vi "main 0.5.vi"() -> ()   [LabVIEW 2015]
uses:
  subvi/PHOIBOS/DEFINITIONS/DEF_dev_state.ctl
  subvi/PHOIBOS/DEFINITIONS/DEF_dev_type.ctl
  <vilib>/Utility/file.llb/Write Delimited Spreadsheet (I64).vi
  subvi/Newport ESP301/Newport ESP301.lvlib
  subvi/sp_manip.llb/sp_manip_lib.lvlib
  subvi/sp_manip.llb/tcp_gateway.lvlib
panel:
  out "appended path 2":path=path "W:/Labview/Front ends/ARPEScontrol/t0.txt"
  out "appended path":path=path "W:/Labview/Front ends/ARPEScontrol/runnumber.txt"
  out "RunNumber":u16=4
  out "# elements in queue":i32
  out "sum":dbl=3886353.0
  out "cam_fps":dbl(slide)=19.67681433793903 caption="FPS" scale=0.1..50.0
  out "max value":u32=54
  out "Intensity Graph":u32[][](graph)
  out "ESP_con?":bool=TRUE caption="ESP301"
  out "phoib_con?":bool caption="PHOIBOS"
  out "manip_con?":bool caption="manipulator"
  out "cam_con?":bool caption="camera"
  in  "main_close":bool
  in  "Tab Control":T1(tab)
  in  "ESP_delta":dbl caption="relative [mm]"
  in  "ESP_-":bool
  in  "ESP_+":bool
  in  "ESP_go":bool
  in  "ESP_dest_t":dbl caption="Delay [fs]"
  in  "ESP_dest":dbl=33.3075 caption="Position [mm]"
  in  "ESP_set_t0":bool
  in  "phoib_I_6s":dbl=3200.0
  in  "phoib_I_5s":dbl=1400.0
  in  "phoib_I_4s":dbl=4.2
  in  "phoib_I_3s":dbl
  in  "phoib_I_2s":dbl=35.0
  in  "phoib_I_1s":dbl=21.9
  in  "phoib_standby":bool
  in  "phoib_set":bool
  out "phoib_I_6":dbl caption="Screen Voltage"
  out "phoib_I_5":dbl caption="Detctor Voltage"
  out "phoib_I_4":dbl caption="Work Function"
  out "phoib_I_3":dbl caption="Coil Current"
  out "phoib_I_2":dbl caption="Pass Energy"
  out "phoib_I_1":dbl caption="Kinetic Energy"
  out "Saved Positions":string[][](table)=[["ertwertwert", "-2.299945", "-2.030214", "38.900024", "50.000762", "0.000887", "-97.998082"], ["uztgugt", "-14.999451", "-13.638894", "442.380066", "13.998380", "-1.893758", "-76.305838"], ["asdf", "-14.999451", "-13.638894", "442.380066", "13.998380", "-1.893758", "-76.305838"], ["test3", "-14.999451", "-13.638894", "441.380066", "13.998380", "-1.893758", "-76.305838"]]
  in  "Save Pos":bool
  in  "Load":bool
  in  "Delete":bool
  in  "ManipRel":dbl=1.0
  in  "ManipRel +":bool
  in  "ManipRel -":bool
  in  "manip.rel.select":enum32{"x", "y", "z", "polar", "tilt", "azimut"}(radio)=enum."polar"
  in  "Move Abs":bool
  in  "stop manip":bool
  in  "dest":dbl[](array[numeric])=[0.007141549166819264, -0.009888298846365134, 431.30615234375, 89.00040512814502, 1.109125024699864, -227.9162918846475] caption="destinations" format="%#.5g"
  out "names":string[](array[string])=["x", "y", "z", "polar", "tilt", "azimut"]
  out "pos":dbl[](array[numeric])=[0.007141549166819264, -0.009888298846365134, 431.30615234375, 89.00040512814502, 1.109125024699864, -227.9162918846475] caption="positions" format="%.5f"
  in  "Mode":T2(ring)=enum."WideAngleMode"
  in  "VoltageRange":enum16{"3.5kV", "1.5kV", "400V", "100V", "10V"}(ring)=enum."400V"
  out "ESP_pos":dbl=33.3075 caption="Position"
  out "ESP_delay":dbl caption="Delay"
  out "ESP_t0":dbl=33.3075 caption="Time Zero @"
  out "phoib_I_7":dbl caption="Conversion Voltage"
  in  "phoib_I_7s":dbl
  in  "phoib_I_8s":dbl
  in  "phoib_I_9s":dbl
  out "phoib_I_8":dbl caption="FD1"
  out "phoib_I_9":dbl caption="FD2"
  out "electronics temp [°C]":i32=30
  out "CCD temp [°C]":i32=-13
  in  "gain":bool
  in  "exposure [ms]":u32=20
  in  "binning":u16(ring)=2 items=["X 1", "X 2", "X 4", "X 8"]
  in  "cam_dark?":bool caption="subtract dark?"
  in  "cam_dark":bool
  in  "cam_dark#":u32 max=1000
  in  "cam_burst":bool
  in  "cam_burstnr":u32 max=100000
  out "cam_burst_progress":i32(slide) scale=0.0..500.0
  in  "delscan_picspstep":u16=1 caption="pics/step" min=1 step=1
  in  "delscan_abort":bool
  out "delscan_progress":u32(slide) scale=0.0..20.0
  in  "delscan_go":bool
  out "delscan_pos":dbl caption="current delay [fs]"
  in  "delscan_end":dbl caption="end [fs]"
  in  "delscan_stepsize":dbl caption="stepsize [fs]"
  in  "delscan_start":dbl caption="start [fs]"
  in  "comment":string
  in  "Radio Buttons":enum32{"Radio Selection 1", "Radio Selection 2"}(radio)
  out "opti_frames":dbl=25.0 caption="#steps_opti"
  out "opti_current_frame":i32=25
  out "Measurement Progress":u8(slide) scale=0.0..100.0
  out "Camera Aquisition":u8(slide) scale=0.0..100.0
  in  "Optimize":bool
  in  "OptiStepSize":dbl=-1.0 caption="Step Size"
  in  "OptiRange":dbl=25.0 caption="Range"
  in  "meas_axis":string(combo)="tilt" caption="Axis"
  in  "meas_avg":i32=60 caption="Frames2Average"
  in  "OptiCancel":bool
  out "#steps_opti":dbl=25.0
  out "current_step_opti":i32=25
  out "ETA":string
  in  "BasePath":path=path "Z:/PESdata"
  in  "Path":path=path "Z:/software/ManipulatorControl/save.txt"
  in  "ROI Bottom":i32=32
  in  "ROI Top":i32=1
  in  "ROI Right":i32=40
  in  "ROI Left":i32=1
  in  "ESP Axis":i32=1 min=1 max=3
  in  "manip_init":bool
  in  "manip_release":bool
  in  "phoib_init":bool
  in  "phoib_release":bool
  in  "ESP_init":bool
  in  "ESP_release":bool
  in  "ESP301 VISA":refnum<visa-resource-name>="COM8"
  in  "cam_boardnr":i32
  in  "cam_init":bool
  in  "cam_release":bool
  out "error out":errorcluster
  out "error out 2":errorcluster
  out "state":T3 items=["Off"=-1, "Standby"=0, "On"=1]
  # "step _ of _"
  # "step _ of _"
  # "manip"
  # "phoib"
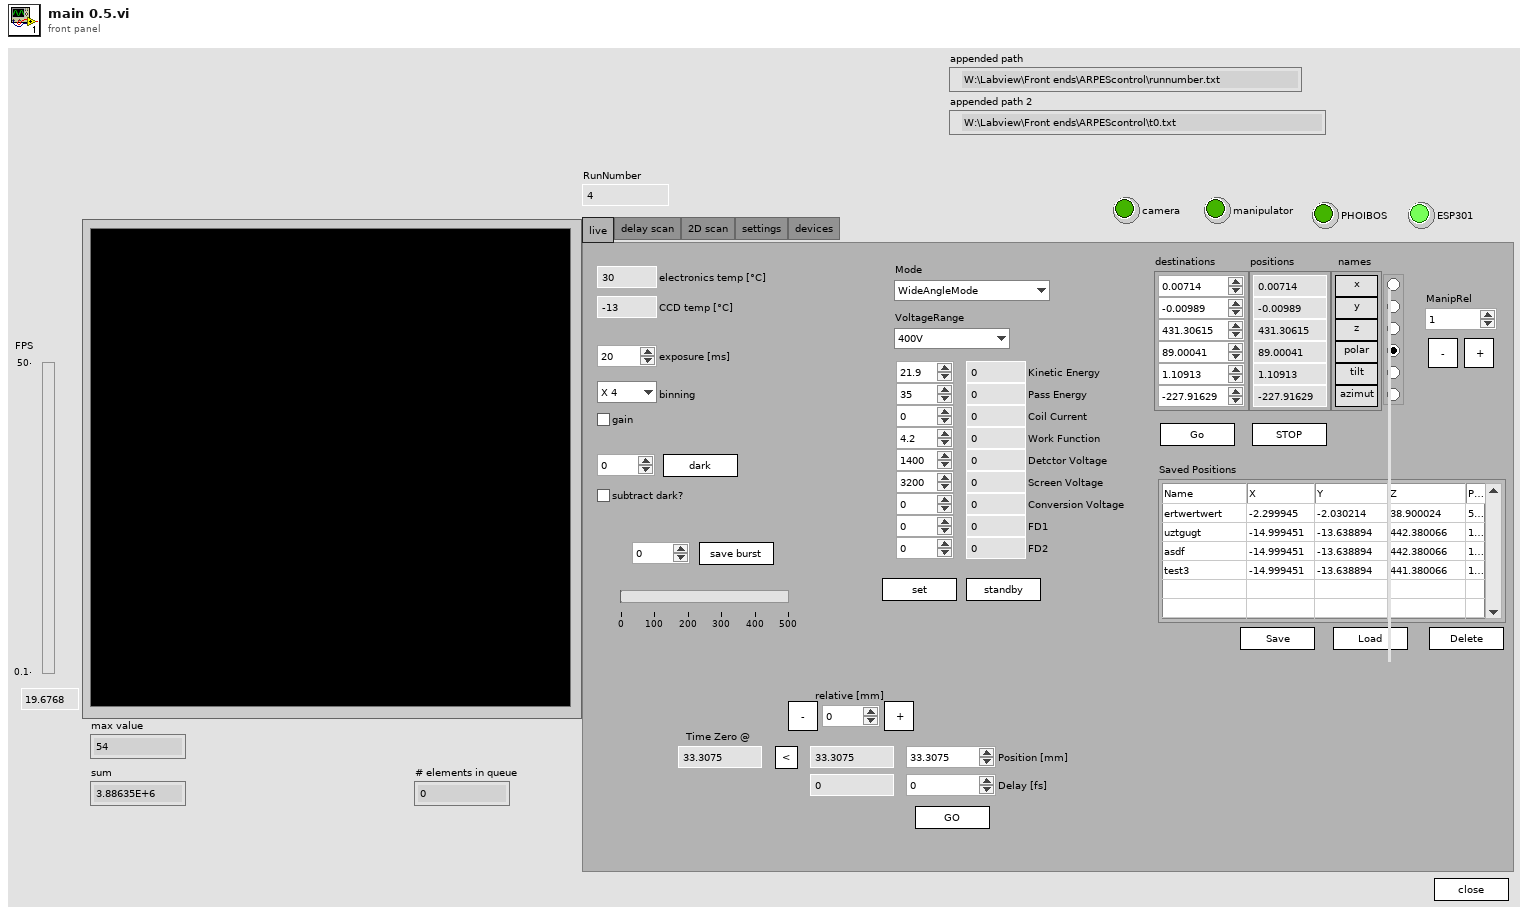
[diagram p1: front panel]
types:
  T1 = enum32{"live", "delay scan", "2D scan", "settings", "devices"}
  T2 = enum16{"HighMagnification", "MediumMagnification", "LowMagnification", "HighAngularDispersion", "MediumAngularDispersion", "LowAngularDispersion", "WideAngleMode", "LargeArea", "MediumArea", "SmallArea", "HighMagnification2", "SmallArea2", "ImagingMode"}
  T3 = typedef "DEF_dev_state.ctl" = i32
  T4 = cluster{"Camera type":u32, "Operating mode\nHP & QE / HS & DiCam Pro ":u32, "Frame trigger \n(High Performance and QE only)":u16, "Sequence trigger":u16, "Low Light\n(QE only)":bool, "Gain":bool, "Horzontal\nbinning":u16, "Vertical\nbinning ":u16, "ROI Left":i32, "ROI Right":i32, "ROI Top":i32, "ROI Bottom":i32}
  T5 = enum16{"open", "replace", "create", "open or create", "replace or create", "replace or create with confirmation"}
  T6 = cluster{"Axis_Name":string, "Axis_Type":string, "Axis_Position":dbl, "continous":bool, "moving":bool}[]
  T7 = cluster{"Axis_Name":string, "Axis_Type":string, "Axis_Position":dbl, "continous":bool, "moving":bool}
  T8 = typedef "DEF_dev_type.ctl" = enum32{"devA (analyzer)", "devD (detector)"}
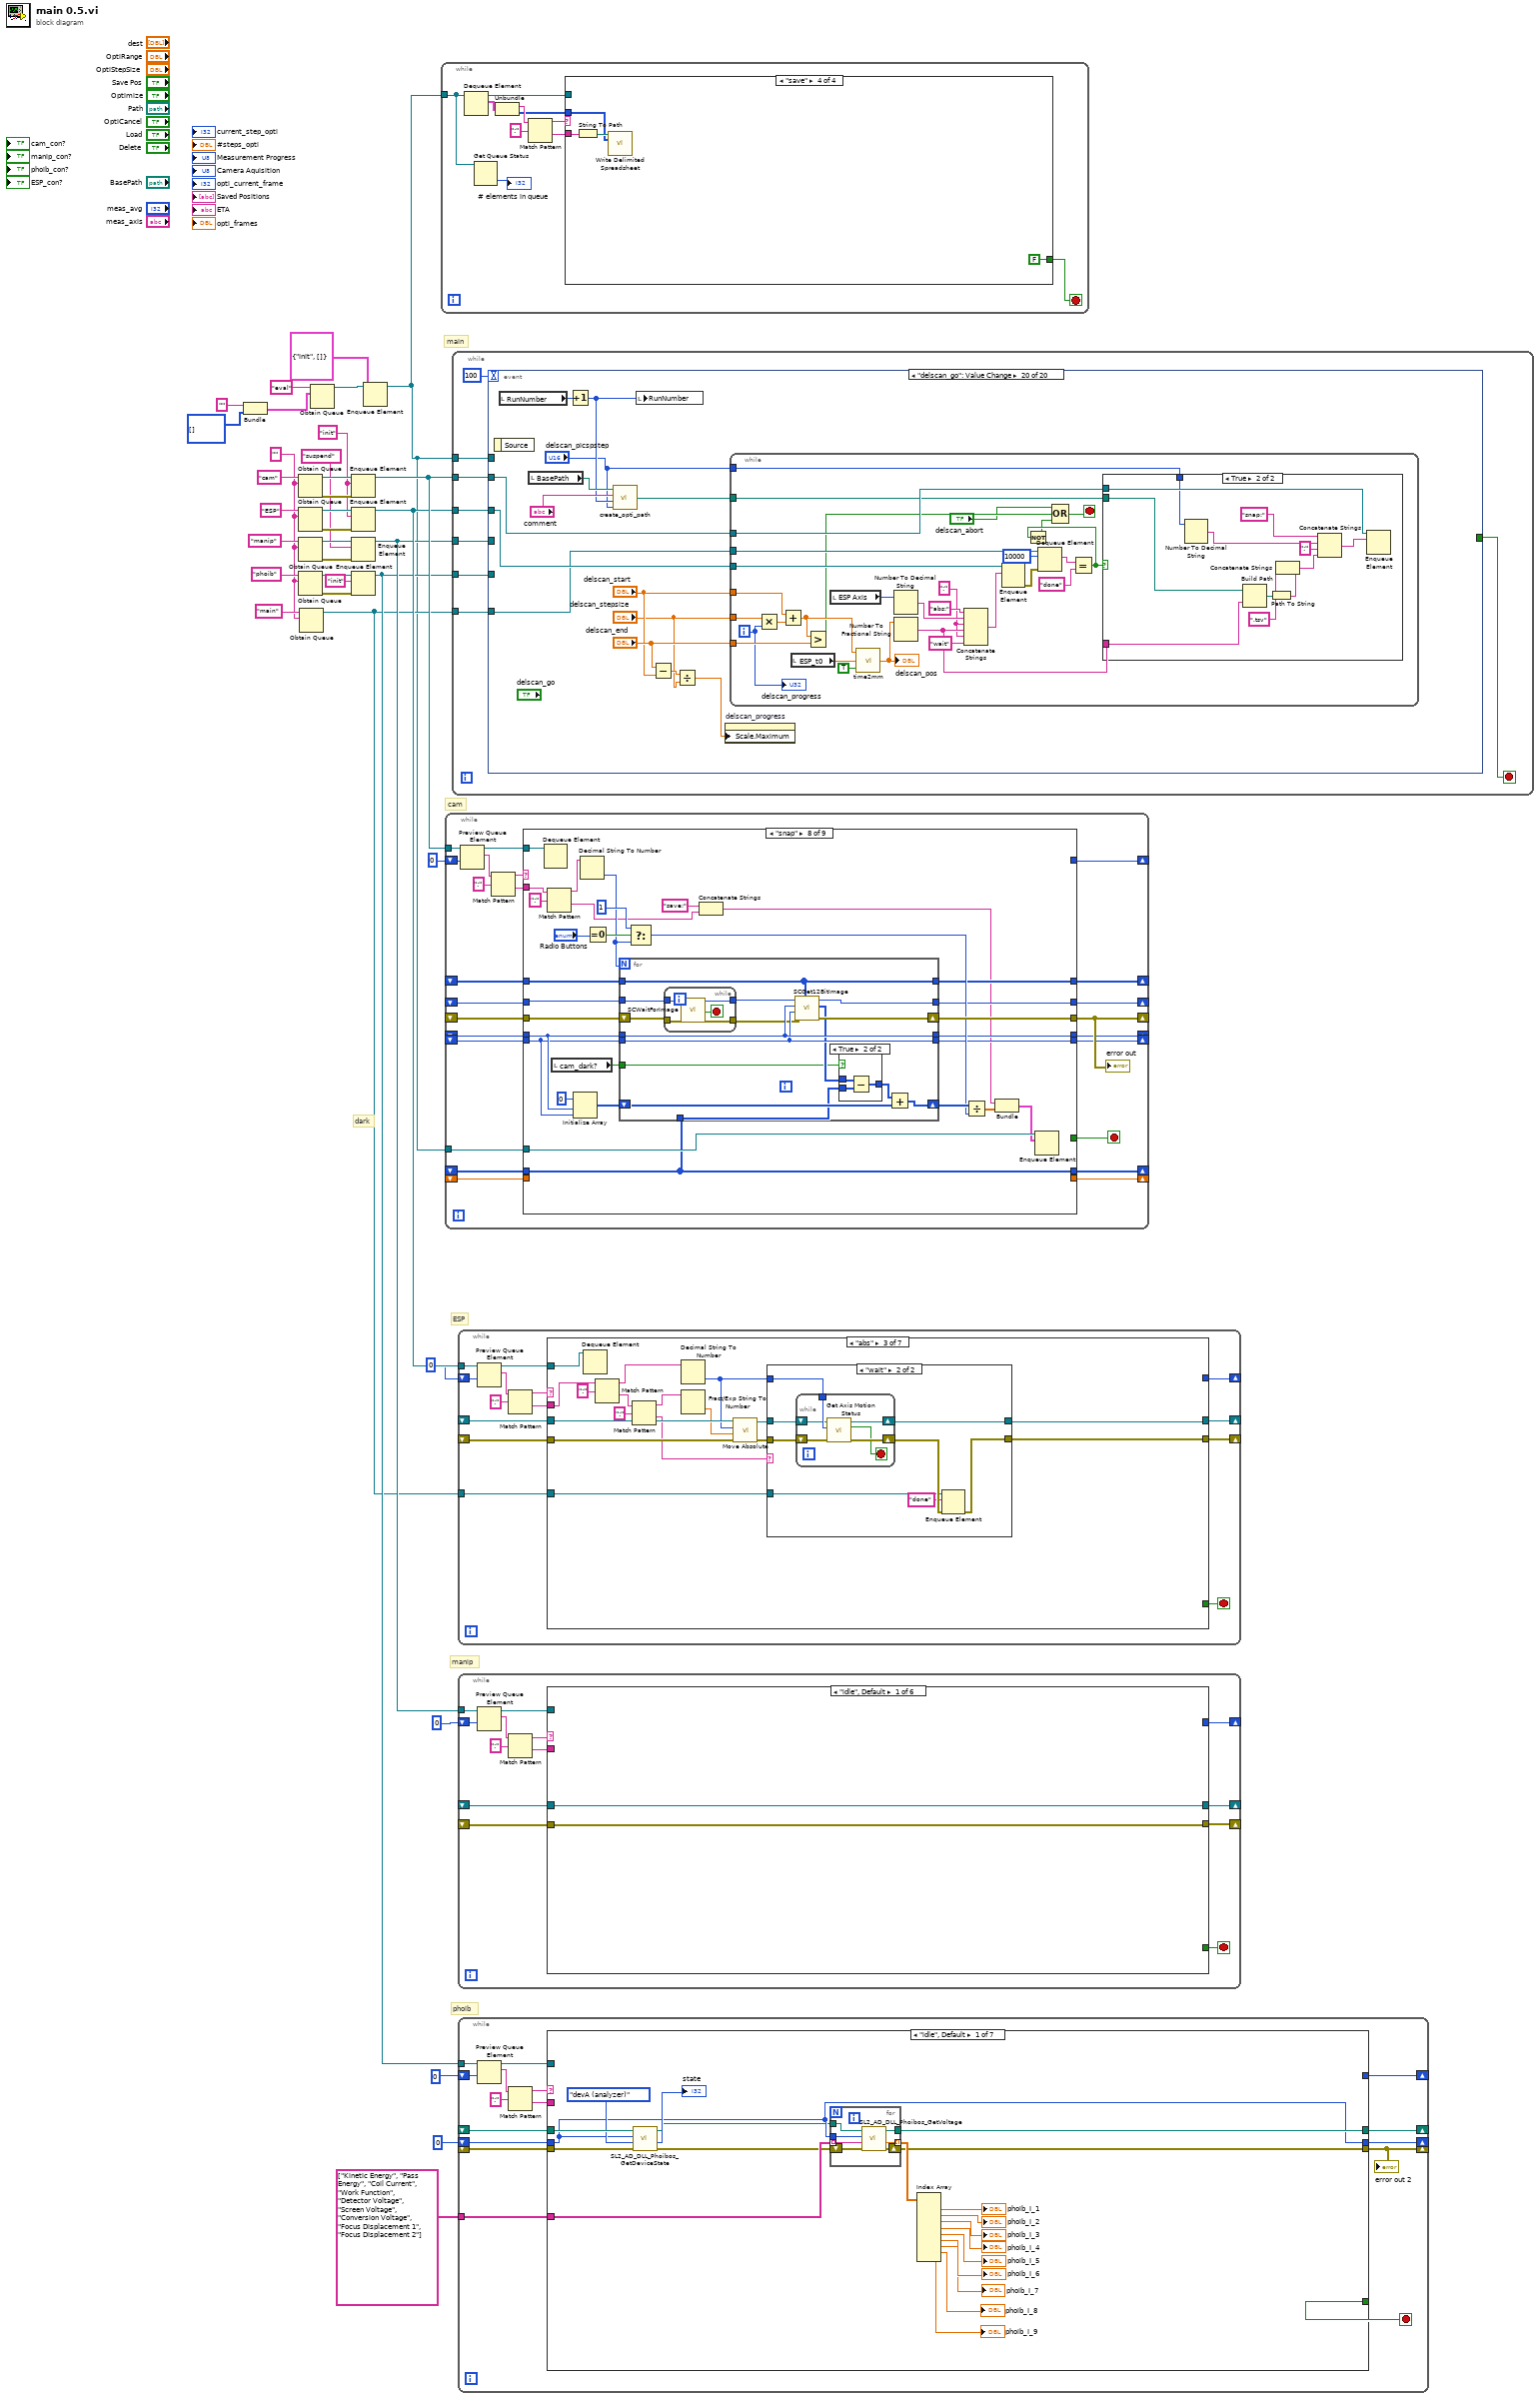
[diagram p0: block diagram]
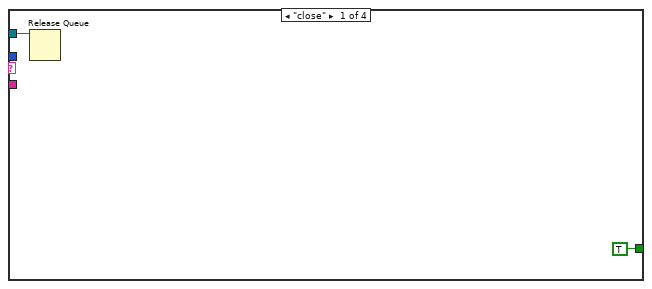
[diagram p2: hidden frame]
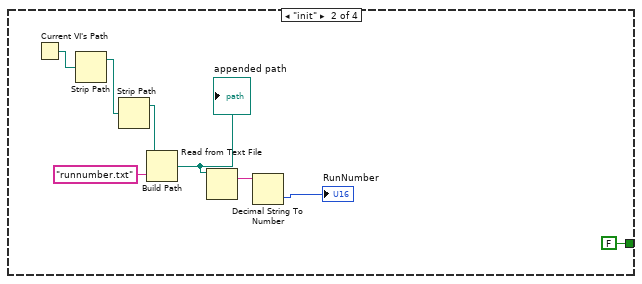
[diagram p3: hidden frame]
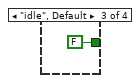
[diagram p4: hidden frame]
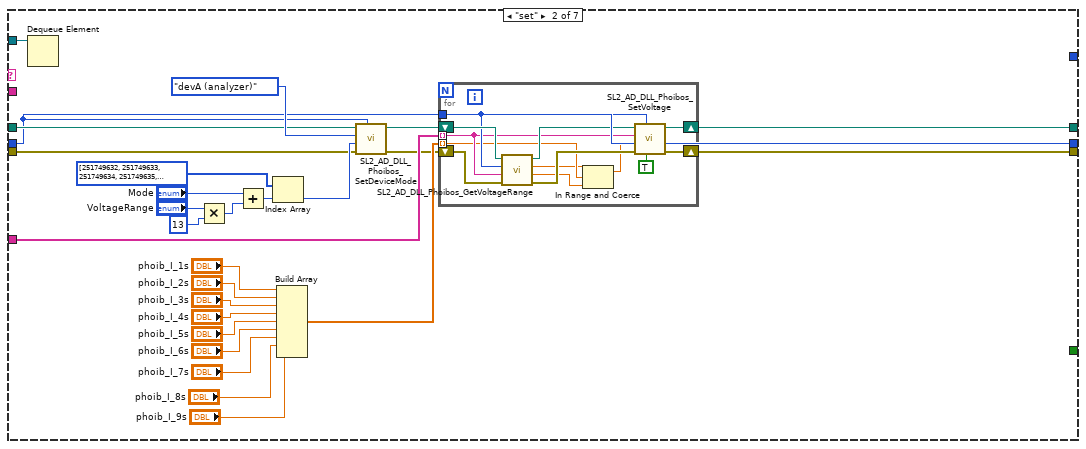
[diagram p5: hidden frame]
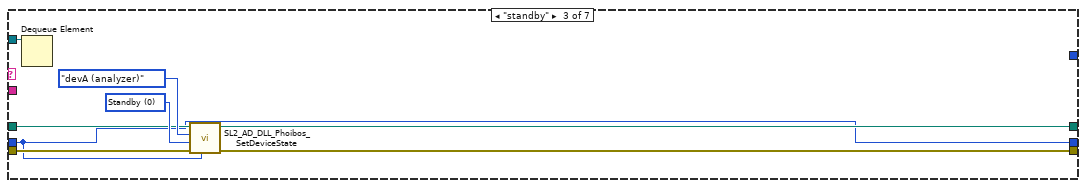
[diagram p6: hidden frame]
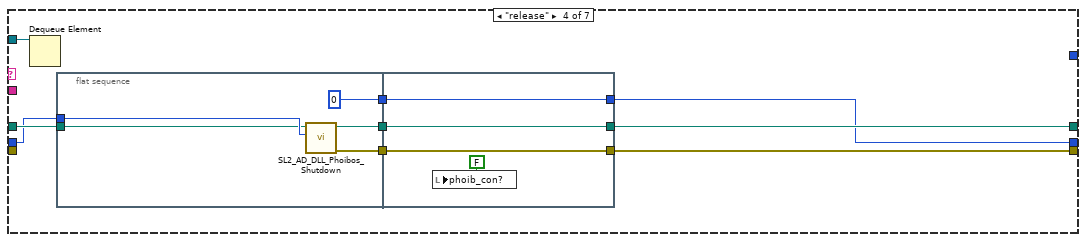
[diagram p7: hidden frame]
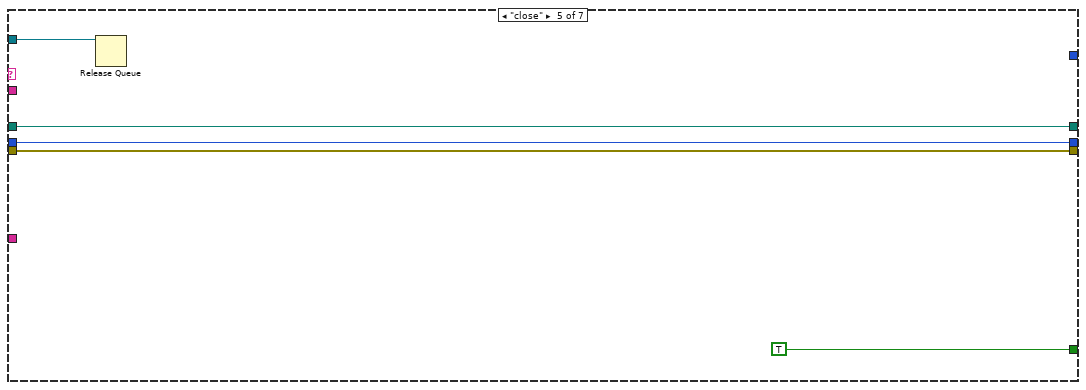
[diagram p8: hidden frame]
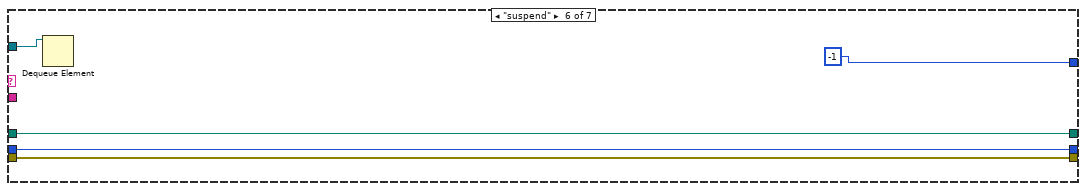
[diagram p9: hidden frame]
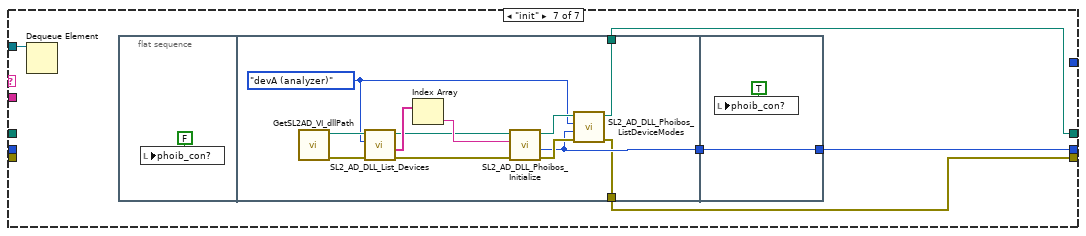
[diagram p10: hidden frame]
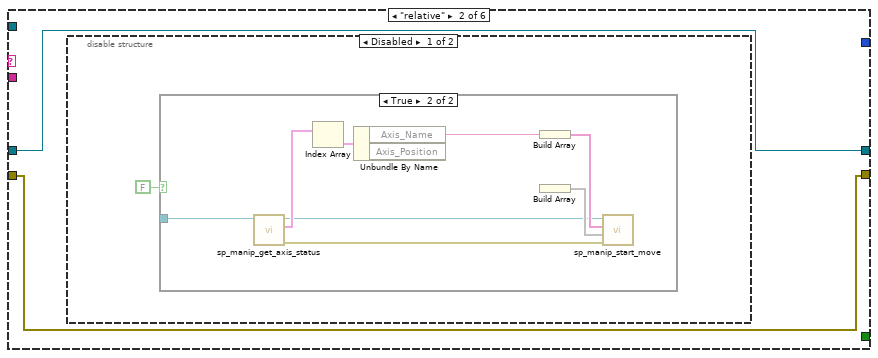
[diagram p11: hidden frame]
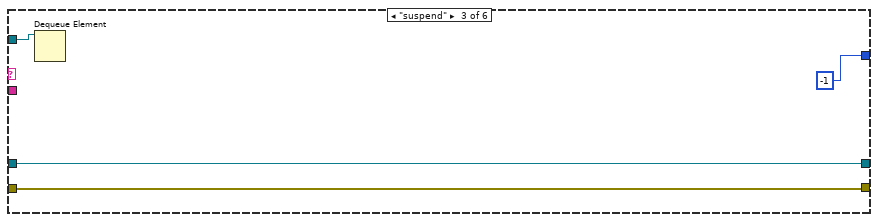
[diagram p14: hidden frame]
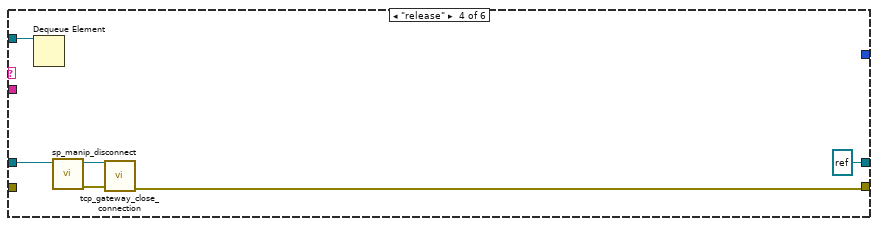
[diagram p15: hidden frame]
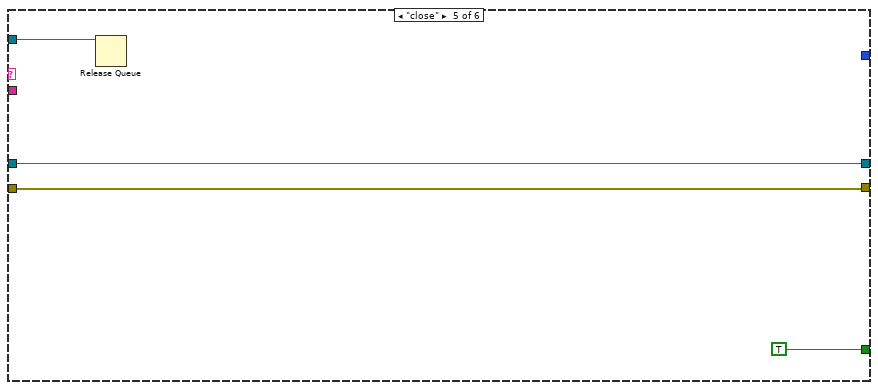
[diagram p16: hidden frame]
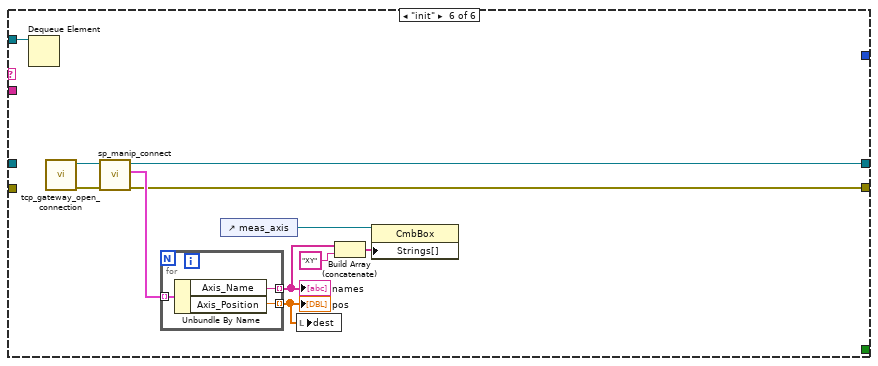
[diagram p17: hidden frame]
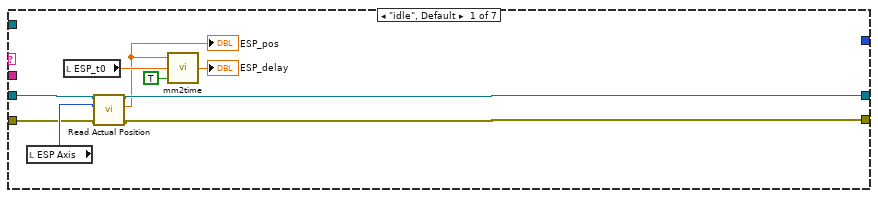
[diagram p18: hidden frame]
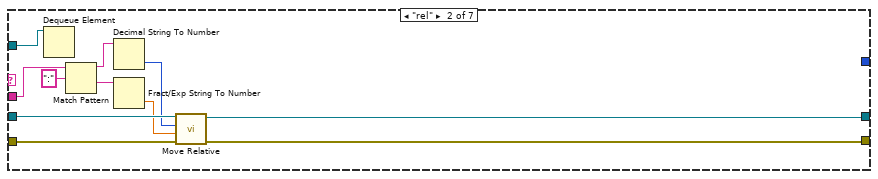
[diagram p19: hidden frame]
diagram:
  w4 = "init" ("name (unnamed)")
  w9 = "" ("name (unnamed)")
  # "dark"
  # "phoib"
  # "manip"
  # "ESP"
  # "cam"
  # "main"
  n1 = Bundle("", u32[][] []) -> (w7:cluster{string, u32[][]})  [unwired: 1 in]
  n2 = Obtain Queue(name (unnamed)="cam", element data type=w9) -> (queue out=w34:refnum<queue>, error out=w33:errorcluster)  [unwired: 3 in, 1 out]
  n3 = Obtain Queue(name (unnamed)="ESP", element data type=w9) -> (queue out=w30:refnum<queue>, error out=w31:errorcluster)  [unwired: 3 in, 1 out]
  n4 = Obtain Queue(name (unnamed)="manip", element data type=w9) -> (queue out=w27:refnum<queue>, error out=w26:errorcluster)  [unwired: 3 in, 1 out]
  n5 = Obtain Queue(name (unnamed)="phoib", element data type=w9) -> (queue out=w24:refnum<queue>, error out=w25:errorcluster)  [unwired: 3 in, 1 out]
  n6 = Obtain Queue(name (unnamed)="main", element data type=w9) -> (queue out=w10:refnum<queue>)  [unwired: 3 in, 2 out]
  n7 = Obtain Queue(name (unnamed)="eval", element data type=w7) -> (queue out=w3:refnum<queue>)  [unwired: 3 in, 2 out]
  n8 = Enqueue Element(queue=w34, element=w4, error in (no error)=w33) -> (queue out=w32:refnum<queue>)  [unwired: 1 in, 2 out]
  n9 = Enqueue Element(queue=w30, element=w4, error in (no error)=w31) -> (queue out=w21:refnum<queue>)  [unwired: 1 in, 2 out]
  n10 = Enqueue Element(queue=w27, element="suspend" ("name (unnamed)"), error in (no error)=w26) -> (queue out=w20:refnum<queue>)  [unwired: 1 in, 2 out]
  n11 = Enqueue Element(queue=w24, element="init", error in (no error)=w25) -> (queue out=w19:refnum<queue>)  [unwired: 1 in, 2 out]
  n12 = Enqueue Element(queue=w3, element=cluster{string, u32[][]} {"init", []}) -> (queue out=w2:refnum<queue>)  [unwired: 2 in, 2 out]
  n13 = while {
    tunnel: w2 -> [w37]
    stop <- w38 stop-if-true
    n14 = Dequeue Element(queue=w37) -> (queue out=w43:refnum<queue>, element=w42:cluster{string, u32[][]})  [unwired: 2 in, 2 out]
    n15 = Get Queue Status(queue=w37) -> (# elements in queue=→"# elements in queue":i32)  [unwired: 2 in, 7 out]
    n16 = Unbundle(w42) -> (w41:string, w40:u32[][])
    n17 = Match Pattern(string=w41, regular expression=":") -> (before substring=w44:string, after substring=w39:string)  [unwired: 1 in, 2 out]
    n18 = case shown="\"save\"" w44 {
      tunnel: w43 -> [w47 _ _ _]
      tunnel: w40 -> [_ _ _ w58]
      tunnel: w39 -> [_ _ _ w60]
      tunnel: [TRUE FALSE FALSE FALSE] -> w38
      frame "close" {
        n19 = Release Queue(queue=w47) -> ()  [unwired: 2 in, 3 out]
      }
      frame "init" {
        n20 = Current VI's Path() -> (path=w55:path)
        n21 = Strip Path(path=w55) -> (stripped path=w49:path)  [unwired: 1 out]
        n22 = Strip Path(path=w49) -> (stripped path=w48:path)  [unwired: 1 out]
        n23 = Build Path(base path=w48, name or relative path="runnumber.txt") -> (appended path=w53:path)
        "appended path" <- w53
        n24 = Read from Text File(file (use dialog)=w53) -> (text=w52:string)  [unwired: 3 in, 3 out]
        n25 = Decimal String To Number(string=w52) -> (number=→"RunNumber":i32)  [unwired: 2 in, 1 out]
      }
      frame "idle", Default {
      }
      frame "save" {
        n26 = String To Path(string=w60) -> (path=w59:path)
        n27 = call-poly <vilib>:"Write Delimited Spreadsheet.vi"("file path (dialog if empty)"=w59, "2D data"=w58) -> ()  [unwired: 12 in, 2 out]
      }
    }
  }
  n28 = while {
    tunnel: w32 -> [w84]
    shift-right: [w78] -> _
    shift-left: _ -> [w77]
    shift-right: [w76] -> _
    shift-left: _ -> [w72]
    shift-right: [w75] -> _
    shift-left: _ -> [w71]
    shift-right: [w74] -> _
    shift-left: _ -> [w70]
    shift-right: [w73] -> _
    shift-left: _ -> [w69]
    shift-right: [w66] -> _
    shift-left: 0 -> [w67]
    shift-right: [w65] -> _
    shift-left: _ -> [w64]
    shift-right: [w63] -> _
    shift-left: _ -> [w62]
    tunnel: w2 -> [w61]
    stop <- w68 stop-if-true
    n29 = Preview Queue Element(queue=w84, timeout in ms (-1)=w67) -> (queue out=w83:refnum<queue>, element=w82:string)  [unwired: 1 in, 2 out]
    n30 = Match Pattern(string=w82, regular expression=":") -> (before substring=w79:string, after substring=w80:string)  [unwired: 1 in, 2 out]
    n31 = case shown="\"snap\"" w79 {
      tunnel: w83 -> [w93 w121 w151 w205 w217 _ w257 w286 w346]
      tunnel: w80 -> [_ _ w159 _ _ _ _ w290 _]
      tunnel: [w87 w110 w148 w204 w215 w241 w255 w302 w344] -> w78
      tunnel: w77 -> [_ _ w156 w204 w215 w241 w262 w310 w344]
      tunnel: [w92 w122 w149 u64 0 ("Hout") w214 w232 w261 w299 w343] -> w76
      tunnel: [w94 w123 w150 w199 w213 w235 w256 w309 w342] -> w75
      tunnel: [w86 w114 w147 w203 w212 w240 w254 w301 w341] -> w74
      tunnel: [w86 w113 w146 w202 w211 w239 w253 w300 w340] -> w73
      tunnel: w72 -> [_ w125 w155 w201 w214 w231 w263 w285 w343]
      tunnel: w71 -> [_ w124 w152 _ w213 w230 w260 w313 w342]
      tunnel: w70 -> [_ _ w154 w203 w212 w240 w259 w308 w341]
      tunnel: w69 -> [_ _ w153 w202 w211 w239 w258 w307 w340]
      tunnel: [_ _ _ _ TRUE _ _ _ _] -> w68
      tunnel: [_ _ _ _ _ _ _ _ -1] -> w66
      tunnel: [w85 w107 _ _ _ w227 _ _ _] -> w65
      tunnel: w64 -> [w85 w107 _ _ _ w226 _ _ _]
      tunnel: [w87 w109 w145 w197 w210 w221 w251 w293 w339] -> w63
      tunnel: w62 -> [_ w109 w145 w197 w210 w221 _ w293 w339]
      tunnel: w61 -> [_ _ w143 _ _ _ _ w298 _]
      frame "init" {
        w86 = 0 ("Horizontal size")
        w87 = u16[][] []
        n32 = flat-sequence {
          tunnel: [w96] -> w91
          tunnel: [w97] -> w90
          tunnel: [w105] -> w92
          tunnel: [w106] -> w94
          tunnel: w91 -> [w106]
          tunnel: w90 -> [w105]
          frame #0 {
            n33 = local write "cam_con?"(FALSE ("cam_con?")) -> ()
          }
          frame #1 {
            n34 = call "SCInitBoard.vi"("boardnr"="cam_boardnr") -> ("Hout"=w100:u32, "error out"=w101:errorcluster)  [unwired: 1 in, 1 out]
            n35 = call "SCSetupCamera.vi"("Handle"=w100, "error in (no error)"=w101) -> ("Hout"=w102:u64, "error out"=w103:errorcluster)  [unwired: 1 out]
            n36 = call "SCStopCOC.vi"("error in (no error)"=w103, "Stop mode"=0, "Handle"=w102) -> ("error out"=w96:errorcluster, "Hout"=w97:u64)
          }
          frame #2 {
            n37 = local write "cam_con?"(TRUE ("cam_con?")) -> ()
          }
        }
        n38 = Dequeue Element(queue=w93) -> (queue out=w89:refnum<queue>)  [unwired: 2 in, 3 out]
        n39 = Enqueue Element At Opposite End(queue=w89, element="set") -> ()  [unwired: 2 in, 3 out]
      }
      frame "set" {
        w120 = u32 1 ("Operating mode\nHP & QE / HS & DiCam Pro")
        n40 = Dequeue Element(queue=w121) -> ()  [unwired: 2 in, 4 out]
        n41 = Bundle By Name(cluster=cluster{"Delay":dbl, "Exposure ":dbl} {"Delay"=0.0, "Exposure "=0.0} ("Delay and exposure"), "Exposure"="exposure [ms]") -> (w117:cluster{"Delay":dbl, "Exposure ":dbl})
        n42 = call "SCStopCOC.vi"("error in (no error)"=w124, "Stop mode"=0, "Handle"=w125) -> ("error out"=w140:errorcluster, "Hout"=w139:u64)
        n43 = Bundle By Name(cluster=T4 {"Camera type"=0, "Operating mode\nHP & QE / HS & DiCam Pro "=0, "Frame trigger \n(High Performance and QE only)"=0, "Sequence trigger"=0, "Low Light\n(QE only)"=FALSE, "Gain"=FALSE, "Horzontal\nbinning"=0, "Vertical\nbinning "=0, "ROI Left"=1, "ROI Right"=20, "ROI Top"=1, "ROI Bottom"=15} ("Camera controls"), "Operating mode\nHP & QE / HS & DiCam Pro"=w120, "Horzontal\nbinning"="binning", "Vertical\nbinning"="binning", "ROI Left"="ROI Left", "ROI Right"="ROI Right", "ROI Top"="ROI Top", "ROI Bottom"="ROI Bottom", "Gain"="gain") -> (w135:T4)
        n44 = call "New delay and exposure forma.vi"("Operating mode\nHP & QE / HS & DiCam Pro"=w120, "Delay and exposure"=w117) -> ("Output table"=w136:string)  [unwired: 3 in]
        n45 = call "SCSetCoC.vi"("error in (no error)"=w140, "Delay and exposure table"=w136, "Camera controls"=w135, "Handle"=w139) -> ("error out"=w128:errorcluster, "Hout"=w127:u64)  [unwired: 1 out]
        n46 = call "SCGetImageSize.vi"("Handle"=w127, "error in (no error)"=w128) -> ("Hout"=w126:u64, "error out"=w108:errorcluster, "Horizontal size"=w114:i32, "Vertical size"=w113:i32)  [unwired: 2 out]
        n47 = Greater?(x=w114, y=w113) -> (0:w115:bool)
        n48 = Initialize Array(u16 0 ("dimension size"), w113, w114) -> (w110:u16[][])
        n49 = call "SCRun.vi"("error in (no error)"=w108, "Run mode"=0, "Handle"=w126) -> ("error out"=w123:errorcluster, "Hout"=w122:u64)  [unwired: 1 out]
        n50 = Select(t=w114, s=w115, f=w113) -> (s? t:f=w112:i32)
        n51 = property on="Intensity Graph" class="IntGraph (strict)"("XScale.Maximum"=w112, "YScale.Maximum"=w112) -> ()  [unwired: 2 in, 2 out]
      }
      frame "burst" {
        n52 = Match Pattern(string=w159, regular expression=":") -> (before substring=w158:string, after substring=w157:string)  [unwired: 1 in, 2 out]
        n53 = Dequeue Element(queue=w151) -> ()  [unwired: 2 in, 4 out]
        n54 = String To Path(string=w157) -> (path=w141:path)
        n55 = Decimal String To Number(string=w158) -> (number=w144:i32)  [unwired: 2 in, 1 out]
        n56 = property on="cam_burst_progress" class="Slide (strict)"("Scale.Maximum"=w144) -> ()  [unwired: 2 in, 2 out]
        n57 = for {
          N: w144 -> [_]
          tunnel: w156 -> [w177]
          tunnel: w155 -> [w186]
          tunnel: w154 -> [w176]
          tunnel: w153 -> [w175]
          tunnel: w145 -> [w181]
          tunnel: [w179] -> w149
          shift-right: [w178] -> w150
          shift-left: w152 -> [w185]
          tunnel: [w177] -> w148
          tunnel: [w176] -> w147
          tunnel: [w175] -> w146
          tunnel: w143 -> [w174]
          tunnel: 100000 ("x") -> [w167]
          tunnel: w141 -> [w166]
          i -> [w161]
          w187 = 0 items=["Normal", "Upside down"] ("mode")
          n58 = Add(x=w167, y=w161) -> (x+y=w171:i32)
          n59 = while {
            tunnel: [w195] -> w183
            tunnel: [w194] -> w184
            tunnel: w186 -> [w193]
            tunnel: w185 -> [w192]
            stop <- w196 stop-if-true
            n60 = call "SCWaitForImage.vi"("Handle"=w193, "error in (no error)"=w192) -> ("Hout"=w194:u64, "Image Valid"=w196:bool, "error out"=w195:errorcluster)  [unwired: 15 in]
          }
          n61 = Number To Decimal String(number=w171) -> (decimal integer string=w170:string)  [unwired: 1 in]
          n62 = String Subset(string=w170, offset (0)=1) -> (substring=w168:string)  [unwired: 1 in]
          n63 = local read "cam_dark?"() -> (w180:bool)
          n64 = Build Path(base path=w166, name or relative path=w168) -> (appended path=w165:path)
          n65 = call "SCGet12BitImage.vi"("mode"=w187, "Input array"=w177, "error in (no error)"=w183, "Vertical size"=w175, "Horizontal size"=w176, "Handle"=w184) -> ("error out"=w178:errorcluster, "imgdata"=w182:u16[][], "Hout"=w179:u64)  [unwired: 1 in]
          n66 = Path To String(path=w165) -> (string=w164:string)
          n67 = Concatenate Strings("save:" ("string"), w164) -> (w163:string)
          n68 = case shown="True" w180 {
            tunnel: w182 -> [w188 w191]
            tunnel: w181 -> [_ w190]
            tunnel: [w188 w189] -> w162
            frame False {
            }
            frame True {
              n69 = Subtract(x=w191, y=w190) -> (x-y=w189:u32[][])
            }
          }
          n70 = local write "Intensity Graph"(w162) -> ()
          n71 = Bundle(w163, "imgdata"=w162) -> (w173:cluster{string, "imgdata":u32[][]})  [unwired: 1 in]
          n72 = Enqueue Element(queue=w174, element=w173) -> ()  [unwired: 2 in, 3 out]
          "cam_burst_progress" <- w161
        }
      }
      frame "release" {
        n73 = Dequeue Element(queue=w205) -> ()  [unwired: 2 in, 4 out]
        n74 = flat-sequence {
          tunnel: w201 -> [w207]
          tunnel: [w206] -> w198
          tunnel: [w209] -> w199
          tunnel: w198 -> [w209]
          frame #0 {
            n75 = call "SCCloseBoard.vi"("Handle"=w207) -> ("error out"=w206:errorcluster)  [unwired: 1 in, 2 out]
          }
          frame #1 {
            n76 = local write "cam_con?"(FALSE ("cam_con?")) -> ()
          }
        }
      }
      frame "close" {
        n77 = Release Queue(queue=w217) -> ()  [unwired: 2 in, 3 out]
      }
      frame "idle", Default {
        w238 = 0 items=["Normal", "Upside down"] ("mode")
        n78 = call <vilib>:"High Resolution Relative Seconds.vi"() -> ("relative seconds"=w227:dbl)
        n79 = while {
          tunnel: [w249] -> w228
          tunnel: [w248] -> w229
          tunnel: w231 -> [w247]
          tunnel: w230 -> [w246]
          stop <- w250 stop-if-true
          n80 = call "SCWaitForImage.vi"("Handle"=w247, "error in (no error)"=w246) -> ("Hout"=w248:u64, "Image Valid"=w250:bool, "error out"=w249:errorcluster)  [unwired: 15 in]
        }
        n81 = Subtract(x=w227, y=w226) -> (x-y=w225:dbl)
        n82 = Reciprocal(x=w225) -> (1/x=→"cam_fps":dbl)
        n83 = call "SCGet12BitImage.vi"("mode"=w238, "Input array"=w241, "error in (no error)"=w228, "Vertical size"=w239, "Horizontal size"=w240, "Handle"=w229) -> ("error out"=w236:errorcluster, "imgdata"=w222:u16[][], "Hout"=w237:u64)  [unwired: 1 in]
        n84 = case shown="True" "cam_dark?" {
          tunnel: w222 -> [w242 w245]
          tunnel: w221 -> [_ w244]
          tunnel: [w242 w243] -> w219
          frame False {
          }
          frame True {
            n85 = Subtract(x=w245, y=w244) -> (x-y=w243:u32[][])
          }
        }
        "Intensity Graph" <- w219
        n86 = call "SCGetStatus.vi"("Handle"=w237, "error in (no error)"=w236) -> ("Hout"=w232:u64, "Electronics temperature"=→"electronics temp [°C]":i32, "CCD temperature"=→"CCD temp [°C]":i32, "error out"=w235:errorcluster)  [unwired: 2 out]
        n87 = Array Max & Min(array=w219) -> (max value=→"max value":u32)  [unwired: 3 out]
        n88 = Add Array Elements(numeric array=w219) -> (sum=→"sum":u32)
      }
      frame "dark" {
        n89 = Dequeue Element(queue=w257) -> ()  [unwired: 2 in, 4 out]
        n90 = Initialize Array(u32 0, w258, w259) -> (w266:u32[][])
        n91 = for {
          N: "cam_dark#" -> [_]
          tunnel: w259 -> [w269]
          tunnel: w258 -> [w268]
          tunnel: w262 -> [w270]
          shift-right: [w275] -> w265
          shift-left: w266 -> [w276]
          tunnel: w263 -> [w274]
          tunnel: [w272] -> w261
          shift-right: [w271] -> w256
          shift-left: w260 -> [w273]
          tunnel: [w270] -> w255
          tunnel: [w269] -> w254
          tunnel: [w268] -> w253
          n92 = while {
            tunnel: [w283] -> w278
            tunnel: [w282] -> w279
            tunnel: w274 -> [w281]
            tunnel: w273 -> [w280]
            stop <- w284 stop-if-true
            n93 = call "SCWaitForImage.vi"("Handle"=w281, "error in (no error)"=w280) -> ("Hout"=w282:u64, "Image Valid"=w284:bool, "error out"=w283:errorcluster)  [unwired: 15 in]
          }
          n94 = call "SCGet12BitImage.vi"("Input array"=w270, "error in (no error)"=w278, "Vertical size"=w268, "Horizontal size"=w269, "Handle"=w279) -> ("error out"=w271:errorcluster, "imgdata"=w277:u16[][], "Hout"=w272:u64)  [unwired: 2 in]
          n95 = Add(x=w277, y=w276) -> (x+y=w275:u32[][])
        }
        n96 = Divide(x=w265, y="cam_dark#") -> (x/y=w252:dbl[][])
        n97 = To Unsigned Long Integer(number=w252) -> (unsigned 32bit integer=w251:u32[][])
      }
      frame "snap" {
        n98 = Dequeue Element(queue=w286) -> ()  [unwired: 2 in, 4 out]
        n99 = Match Pattern(string=w290, regular expression=":") -> (before substring=w289:string, after substring=w287:string)  [unwired: 1 in, 2 out]
        n100 = local read "cam_dark?"() -> (w292:bool)
        n101 = Initialize Array(u32 0 ("element"), w308, w307) -> (w312:u32[][])
        n102 = Decimal String To Number(string=w289) -> (number=w288:i32)  [unwired: 2 in, 1 out]
        n103 = Equal To 0?(x="Radio Buttons") -> (x = 0?=w303:bool)
        n104 = for {
          N: w288 -> [_]
          tunnel: w308 -> [w325]
          tunnel: w307 -> [w324]
          tunnel: w310 -> [w326]
          shift-right: [w328] -> w311
          shift-left: w312 -> [w329]
          shift-right: [w327] -> w309
          shift-left: w313 -> [w316]
          tunnel: [w326] -> w302
          tunnel: [w325] -> w301
          tunnel: [w324] -> w300
          tunnel: [w323] -> w299
          tunnel: w293 -> [w320]
          tunnel: w292 -> [w319]
          tunnel: w285 -> [w317]
          n105 = while {
            tunnel: [w333] -> w315
            tunnel: [w332] -> w318
            tunnel: w317 -> [w331]
            tunnel: w316 -> [w330]
            stop <- w334 stop-if-true
            n106 = call "SCWaitForImage.vi"("Handle"=w331, "error in (no error)"=w330) -> ("Hout"=w332:u64, "Image Valid"=w334:bool, "error out"=w333:errorcluster)  [unwired: 15 in]
          }
          n107 = call "SCGet12BitImage.vi"("Input array"=w326, "error in (no error)"=w315, "Vertical size"=w324, "Horizontal size"=w325, "Handle"=w318) -> ("error out"=w327:errorcluster, "imgdata"=w321:u16[][], "Hout"=w323:u64)  [unwired: 2 in]
          n108 = case shown="True" w319 {
            tunnel: [w335 w336] -> w322
            tunnel: w321 -> [w335 w338]
            tunnel: w320 -> [_ w337]
            frame False {
            }
            frame True {
              n109 = Subtract(x=w338, y=w337) -> (x-y=w336:u32[][])
            }
          }
          n110 = Add(x=w322, y=w329) -> (x+y=w328:u32[][])
        }
        n111 = Select(t=1, s=w303, f=w288) -> (s? t:f=w306:i32)
        n112 = Concatenate Strings("save:" ("string"), w287) -> (w297:string)
        n113 = Divide(x=w311, y=w306) -> (x/y=w296:dbl[][])
        n114 = Bundle(w297, w296) -> (w295:cluster{string, dbl[][]})  [unwired: 1 in]
        n115 = Enqueue Element(queue=w298, element=w295) -> ()  [unwired: 2 in, 3 out]
      }
      frame "suspend" {
        n116 = Dequeue Element(queue=w346) -> ()  [unwired: 2 in, 4 out]
      }
    }
    "error out" <- w75
  }
  n117 = while {
    tunnel: w32 -> [w352]
    tunnel: w21 -> [w351]
    tunnel: w20 -> [w350]
    tunnel: w19 -> [w349]
    tunnel: w10 -> [w348]
    tunnel: w2 -> [w347]
    stop <- w354 stop-if-true
    n118 = event shown="[19] \"delscan_go\": Value Change" {
      selector: _ -> [_ _ _ _ _ _ _ _ _ _ _ _ _ _ _ _ _ _ _ _]
      dyn-events: _ -> [_ _ _ _ _ _ _ _ _ _ _ _ _ _ _ _ _ _ _ _]
      timeout: 100 -> [_ _ _ _ _ _ _ _ _ _ _ _ _ _ _ _ _ _ _ _]
      tunnel: [_ TRUE _ _ _ _ _ _ _ _ _ _ _ _ _ _ _ _ _ _] -> w354
      tunnel: w352 -> [_ w367 w370 _ _ _ _ _ w396 w398 w399 _ _ _ _ _ _ _ _ w483]
      tunnel: w351 -> [_ w366 _ w374 _ _ _ _ _ _ _ _ _ _ w445 _ w457 _ _ w485]
      tunnel: w350 -> [_ w365 _ _ w380 _ _ _ _ _ _ _ _ _ _ _ _ _ _ _]
      tunnel: w349 -> [_ w364 _ _ _ w386 w392 w393 _ _ _ _ _ _ _ _ _ _ _ _]
      tunnel: w348 -> [_ w357 _ _ _ _ _ _ _ _ _ _ _ _ _ _ _ _ _ w484]
      tunnel: w347 -> [_ w356 _ _ _ _ _ _ _ _ _ _ _ _ _ _ _ _ _ _]
      event Timeout {
        n119 = event-data() -> ()  [unwired: 1 in, 1 out]
      }
      event "main_close": Value Change {
        w358 = "close" ("element")
        w363 = "release" ("element")
        n120 = event-data() -> ()  [unwired: 1 in, 1 out]
        n121 = Enqueue Element(queue=w367, element=w363) -> (queue out=w362:refnum<queue>)  [unwired: 2 in, 2 out]
        n122 = Enqueue Element(queue=w366, element=w363) -> (queue out=w361:refnum<queue>)  [unwired: 2 in, 2 out]
        n123 = Enqueue Element(queue=w365, element=w363) -> (queue out=w360:refnum<queue>)  [unwired: 2 in, 2 out]
        n124 = Enqueue Element(queue=w364, element=w363) -> (queue out=w359:refnum<queue>)  [unwired: 2 in, 2 out]
        n125 = Release Queue(queue=w357) -> ()  [unwired: 2 in, 3 out]
        n126 = Enqueue Element(queue=w362, element=w358) -> ()  [unwired: 2 in, 3 out]
        n127 = Enqueue Element(queue=w361, element=w358) -> ()  [unwired: 2 in, 3 out]
        n128 = Enqueue Element(queue=w360, element=w358) -> ()  [unwired: 2 in, 3 out]
        n129 = Enqueue Element(queue=w359, element=w358) -> ()  [unwired: 2 in, 3 out]
        n130 = Enqueue Element(queue=w356, element=cluster{string, u32[][]} {"close", []}) -> ()  [unwired: 2 in, 3 out]
      }
      event "cam_release", "cam_init": Value Change {
        n131 = event-data() -> ()  [unwired: 1 in, 2 out]
        n132 = Select(t="init" ("name (unnamed)"), s="cam_init", f="release" ("name (unnamed)")) -> (s? t:f=w369:string)
        n133 = Enqueue Element(queue=w370, element=w369) -> ()  [unwired: 2 in, 3 out]
      }
      event "ESP_release", "ESP_init": Value Change {
        n134 = event-data() -> ()  [unwired: 1 in, 2 out]
        n135 = Select(t="init" ("name (unnamed)"), s="ESP_init", f="release" ("name (unnamed)")) -> (s? t:f=w378:string)
        n136 = Enqueue Element(queue=w374, element=w378) -> ()  [unwired: 2 in, 3 out]
      }
      event "manip_init", "manip_release": Value Change {
        n137 = event-data() -> ()  [unwired: 1 in, 2 out]
        n138 = Flush Queue(queue=w380) -> (queue out=w379:refnum<queue>)  [unwired: 1 in, 2 out]
        n139 = Select(t="init" ("name (unnamed)"), s="manip_init", f="release" ("name (unnamed)")) -> (s? t:f=w382:string)
        n140 = Enqueue Element(queue=w379, element=w382) -> ()  [unwired: 2 in, 3 out]
      }
      event "phoib_release", "phoib_init": Value Change {
        n141 = event-data() -> ()  [unwired: 1 in, 2 out]
        n142 = Flush Queue(queue=w386) -> (queue out=w385:refnum<queue>)  [unwired: 1 in, 2 out]
        n143 = Select(t="init" ("name (unnamed)"), s="phoib_init", f="release" ("name (unnamed)")) -> (s? t:f=w388:string)
        n144 = Enqueue Element(queue=w385, element=w388) -> ()  [unwired: 2 in, 3 out]
      }
      event "phoib_standby": Value Change {
        n145 = event-data() -> ()  [unwired: 1 in, 2 out]
        n146 = Enqueue Element(queue=w392, element="standby") -> ()  [unwired: 2 in, 3 out]
      }
      event "phoib_set": Value Change {
        n147 = event-data() -> ()  [unwired: 1 in, 2 out]
        n148 = Enqueue Element(queue=w393, element="set") -> ()  [unwired: 2 in, 3 out]
      }
      event "cam_dark": Value Change {
        n149 = event-data() -> ()  [unwired: 1 in, 2 out]
        n150 = Enqueue Element(queue=w396, element="dark") -> ()  [unwired: 2 in, 3 out]
      }
      event "ROI Left", "ROI Right", "ROI Top", "ROI Bottom", "exposure [ms]", "binning", "gain": Value Change {
        n151 = event-data() -> ()  [unwired: 1 in, 6 out]
        n152 = Enqueue Element(queue=w398, element="set") -> ()  [unwired: 2 in, 3 out]
      }
      event "cam_burst": Value Change {
        n153 = event-data() -> ()  [unwired: 1 in, 1 out]
        n154 = local read "BasePath"() -> (w403:path)
        n155 = call "File Dialog"("start path"=w403) -> ("selected path"=w401:path, "cancelled"=w402:bool, "error out"=w400:errorcluster)  [unwired: 11 in, 1 out]
        n156 = case shown="False" w402 {
          tunnel: w401 -> [w427 _]
          tunnel: w400 -> [_ _]
          tunnel: w399 -> [w434 _]
          frame False {
            w422 = "\r"
            w421 = "\t"
            n157 = local read "exposure [ms]"() -> (w414:u32)
            n158 = local read "binning"() -> (w412:u16)
            n159 = local read "gain"() -> (w413:bool)
            n160 = Boolean To (0,1)(Boolean=w413) -> (0, 1=w411:i16)
            n161 = Number To Decimal String(number=w414) -> (decimal integer string=w409:string)  [unwired: 1 in]
            n162 = Number To Decimal String(number=w411) -> (decimal integer string=w407:string)  [unwired: 1 in]
            n163 = Number To Decimal String(number=w412) -> (decimal integer string=w405:string)  [unwired: 1 in]
            n164 = Get Date/Time In Seconds() -> (seconds since 1Jan1904=w425:timestamp)
            n165 = Format Date/Time String(time format string (%c)="%Y.%m.%d-%H.%M.%S", seconds (now)=w425) -> (date/time string=w424:string)  [unwired: 1 in]
            n166 = Concatenate Strings("Exposure:", w421, w409, w422, "Gain:", w421, w407, w422, "binning", w421, w405, w422) -> (w415:string)
            n167 = Build Path(base path=w427, name or relative path=w424) -> (appended path=w423:path)
            n168 = Create Folder(path (use dialog)=w423) -> (created path=w404:path)  [unwired: 2 in, 2 out]
            n169 = Build Path(base path=w404, name or relative path="info.txt") -> (appended path=w419:path)
            n170 = Number To Decimal String(number="cam_burstnr") -> (decimal integer string=w431:string)  [unwired: 1 in]
            n171 = Path To String(path=w404) -> (string=w429:string)
            n172 = Open/Create/Replace File(file path (use dialog)=w419, operation (0:open)=T5."replace or create") -> (refnum out=w417:refnum<file>)  [unwired: 4 in, 2 out]
            n173 = Write to Text File(file (use dialog)=w417, text=w415) -> (refnum out=w416:refnum<file>)  [unwired: 2 in, 2 out]
            n174 = Close File(refnum=w416) -> ()  [unwired: 1 in, 2 out]
            n175 = Concatenate Strings("burst:" ("string"), w431, ":" ("string"), w429) -> (w428:string)
            n176 = Enqueue Element(queue=w434, element=w428) -> ()  [unwired: 2 in, 3 out]
          }
          frame True {
          }
        }
      }
      event "Move Abs": Value Change {
        n177 = event-data() -> ()  [unwired: 1 in, 1 out]
      }
      event "ManipRel +", "ManipRel -": Value Change {
        n178 = event-data() -> ()  [unwired: 1 in, 2 out]
        n179 = Negate(x="ManipRel") -> (-x=w436:dbl)
        n180 = Select(t=w436, s="ManipRel -", f="ManipRel") -> ()  [unwired: 1 out]
      }
      event "stop manip": Value Change {
        n181 = event-data() -> ()  [unwired: 1 in, 1 out]
      }
      event "ESP_go": Value Change {
        w439 = ":" ("string")
        n182 = event-data() -> ()  [unwired: 1 in, 1 out]
        n183 = local read "ESP Axis"() -> (w438:i32)
        n184 = Number To Decimal String(number=w438) -> (decimal integer string=w441:string)  [unwired: 1 in]
        n185 = Number To Fractional String(number="ESP_dest") -> (F-format string=w440:string)  [unwired: 3 in]
        n186 = Concatenate Strings("abs:" ("string"), w441, w439, w440, w439) -> (w444:string)
        n187 = Enqueue Element(queue=w445, element=w444) -> ()  [unwired: 2 in, 3 out]
      }
      event "ESP_set_t0": Value Change {
        n188 = event-data() -> ()  [unwired: 1 in, 1 out]
        n189 = Current VI's Path() -> (path=w451:path)
        n190 = local read "ESP_pos"() -> (w449:dbl)
        "ESP_t0" <- w449
        n191 = Strip Path(path=w451) -> (stripped path=w447:path)  [unwired: 1 out]
        n192 = Strip Path(path=w447) -> (stripped path=w446:path)  [unwired: 1 out]
        n193 = Number To Fractional String(number=w449) -> (F-format string=w448:string)  [unwired: 3 in]
        n194 = Build Path(base path=w446, name or relative path="t0.txt") -> (appended path=w450:path)
        "appended path 2" <- w450
        n195 = Write to Text File(file (use dialog)=w450, text=w448) -> ()  [unwired: 2 in, 3 out]
      }
      event "ESP_+", "ESP_-": Value Change {
        n196 = event-data() -> ()  [unwired: 1 in, 6 out]
        n197 = Negate(x="ESP_delta") -> (-x=w460:dbl)
        n198 = Select(t="ESP_delta", s="ESP_+", f=w460) -> (s? t:f=w458:dbl)
        n199 = Number To Decimal String(number="ESP Axis") -> (decimal integer string=w455:string)  [unwired: 1 in]
        n200 = Number To Fractional String(number=w458) -> (F-format string=w453:string)  [unwired: 3 in]
        n201 = Concatenate Strings("rel:" ("string"), w455, ":" ("string"), w453) -> (w463:string)
        n202 = Enqueue Element(queue=w457, element=w463) -> ()  [unwired: 2 in, 3 out]
      }
      event "ESP_dest": Value Change {
        n203 = event-data() -> ()  [unwired: 1 in, 6 out]
        n204 = local read "ESP_dest"() -> (w467:dbl)
        n205 = local read "ESP_t0"() -> (w466:dbl)
        n206 = call "mm2time.vi"("fs?"=TRUE ("fs[1]/ps[0]"), "Offset (mm)"=w466, "distance (mm)"=w467) -> ("time in fs/ps seconds"=w464:dbl)
        n207 = local write "ESP_dest_t"(w464) -> ()
      }
      event "ESP_dest_t": Value Change {
        n208 = event-data() -> ()  [unwired: 1 in, 1 out]
        n209 = local read "ESP_t0"() -> (w470:dbl)
        n210 = call "time2mm.vi"("fs[1]/ps[0]"=TRUE, "Offset (mm)"=w470, "time"="ESP_dest_t") -> ("position (mm)"=w468:dbl)
        n211 = local write "ESP_dest"(w468) -> ()
      }
      event "delscan_go": Value Change {
        n212 = event-data() -> ()  [unwired: 1 in, 1 out]
        n213 = local read "RunNumber"() -> (w482:u16)
        n214 = local read "BasePath"() -> (w481:path)
        n215 = Increment(x=w482) -> (x+1=w479:u16)
        n216 = call "create_opti_path.vi"("N"="delscan_picspstep", "RunNumber"=w479, "comment"="comment", "base path"=w481) -> ("Path"=w477:path)
        n217 = local write "RunNumber"(w479) -> ()
        n218 = Subtract(x="delscan_end", y="delscan_start") -> (x-y=w474:dbl)
        n219 = Divide(x=w474, y="delscan_stepsize") -> (x/y=w472:dbl)
        n220 = property on="delscan_progress" class="Slide (strict)"("Scale.Maximum"=w472) -> ()  [unwired: 2 in, 2 out]
        n221 = while {
          tunnel: "delscan_stepsize" -> [w515]
          tunnel: "delscan_start" -> [w513]
          tunnel: "delscan_end" -> [w512]
          tunnel: w485 -> [w504]
          tunnel: w484 -> [w502]
          tunnel: w483 -> [w497]
          tunnel: "delscan_picspstep" -> [w495]
          tunnel: w477 -> [w494]
          i -> [w498]
          stop <- w491 stop-if-true
          w490 = ":" ("string")
          n222 = Multiply(x=w515, y=w498) -> (x*y=w514:dbl)
          n223 = Add(x=w513, y=w514) -> (x+y=w506:dbl)
          n224 = local read "ESP_t0"() -> (w507:dbl)
          n225 = Greater?(x=w506, y=w512) -> (0:w493:bool)
          n226 = local read "ESP Axis"() -> (w505:i32)
          n227 = call "time2mm.vi"("fs[1]/ps[0]"=TRUE, "Offset (mm)"=w507, "time"=w506) -> ("position (mm)"=w503:dbl)
          "delscan_pos" <- w503
          n228 = Number To Decimal String(number=w505) -> (decimal integer string=w509:string)  [unwired: 1 in]
          n229 = Number To Fractional String(number=w503) -> (F-format string=w496:string)  [unwired: 3 in]
          n230 = Concatenate Strings("abs:" ("string"), w509, w490, w496, w490, "wait" ("string")) -> (w511:string)
          n231 = Enqueue Element(queue=w504, element=w511) -> (error out=w501:errorcluster)  [unwired: 2 in, 2 out]
          n232 = Dequeue Element(queue=w502, timeout in ms (-1)=10000, error in (no error)=w501) -> (element=w500:string)  [unwired: 3 out]
          n233 = Equal?(x=w500, y="done") -> (x = y?=w489:bool)
          n234 = Not(x=w489) -> (.not. x?=w488:bool)
          n235 = Compound Arithmetic op=OR("delscan_abort", w493, w488) -> (w491:bool)
          n236 = case shown="True" w489 {
            tunnel: w497 -> [_ w528]
            tunnel: w496 -> [_ w524]
            tunnel: w495 -> [_ w519]
            tunnel: w494 -> [_ w518]
            frame False {
              n237 = One Button Dialog(message="esp error") -> ()  [unwired: 1 in, 1 out]
            }
            frame True {
              n238 = Number To Decimal String(number=w519) -> (decimal integer string=w525:string)  [unwired: 1 in]
              n239 = Build Path(base path=w518, name or relative path=w524) -> (appended path=w522:path)
              n240 = Path To String(path=w522) -> (string=w521:string)
              n241 = Concatenate Strings(w521, ".tsv" ("string")) -> (w523:string)
              n242 = Concatenate Strings("snap:" ("element"), w525, ":" ("string"), w523) -> (w527:string)
              n243 = Enqueue Element(queue=w528, element=w527) -> ()  [unwired: 2 in, 3 out]
            }
          }
          "delscan_progress" <- w498
        }
      }
    }
  }
  n244 = while {
    tunnel: w21 -> [w537]
    shift-right: [w535] -> _
    shift-left: _ -> [w533]
    shift-right: [w534] -> _
    shift-left: _ -> [w532]
    shift-right: [w530] -> _
    shift-left: 0 -> [w531]
    tunnel: w10 -> [w529]
    stop <- w536 stop-if-true
    n245 = Preview Queue Element(queue=w537, timeout in ms (-1)=w531) -> (queue out=w540:refnum<queue>, element=w541:string)  [unwired: 1 in, 2 out]
    n246 = Match Pattern(string=w541, regular expression=":") -> (before substring=w539:string, after substring=w538:string)  [unwired: 1 in, 2 out]
    n247 = case shown="\"abs\"" w539 {
      tunnel: w540 -> [_ w552 w569 w599 w600 w607 w612]
      tunnel: w538 -> [_ w557 w577 _ _ _ _]
      tunnel: [_ _ _ _ _ TRUE _] -> w536
      tunnel: [w544 w559 w570 w597 refnum<visa-resource-name> refnum ("VISA resource name out") w604 w611] -> w535
      tunnel: [w545 w560 w568 w596 w602 w605 w610] -> w534
      tunnel: w533 -> [w548 w562 w575 w597 w603 w604 _]
      tunnel: w532 -> [w546 w561 w576 w596 _ w605 _]
      tunnel: [_ _ _ -1 _ _ _] -> w530
      tunnel: w529 -> [_ _ w567 _ _ _ _]
      frame "idle", Default {
        n248 = local read "ESP Axis"() -> (w547:i32)
        n249 = local read "ESP_t0"() -> (w551:dbl)
        n250 = call "Read Actual Position.vi"("error in (no error)"=w546, "Axis (1)"=w547, "VISA resource name"=w548) -> ("error out"=w545:errorcluster, "Position (units)"=w543:dbl, "VISA resource name out"=w544:refnum<visa-resource-name>)  [unwired: 2 in]
        "ESP_pos" <- w543
        n251 = call "mm2time.vi"("fs?"=TRUE, "Offset (mm)"=w551, "distance (mm)"=w543) -> ("time in fs/ps seconds"=→"ESP_delay":dbl)
      }
      frame "rel" {
        n252 = Dequeue Element(queue=w552) -> ()  [unwired: 2 in, 4 out]
        n253 = Match Pattern(string=w557, regular expression=":") -> (before substring=w556:string, after substring=w555:string)  [unwired: 1 in, 2 out]
        n254 = Decimal String To Number(string=w556) -> (number=w554:i32)  [unwired: 2 in, 1 out]
        n255 = Fract/Exp String To Number(string=w555) -> (number=w553:dbl)  [unwired: 3 in, 1 out]
        n256 = call "Move Relative.vi"("error in (no error)"=w561, "Position (0 units)"=w553, "Axis (1)"=w554, "VISA resource name"=w562) -> ("error out"=w560:errorcluster, "VISA resource name out"=w559:refnum<visa-resource-name>)  [unwired: 2 in]
      }
      frame "abs" {
        n257 = Dequeue Element(queue=w569) -> ()  [unwired: 2 in, 4 out]
        n258 = Match Pattern(string=w577, regular expression=":") -> (before substring=w578:string, after substring=w565:string)  [unwired: 1 in, 2 out]
        n259 = Match Pattern(string=w565, regular expression=":") -> (before substring=w564:string, after substring=w563:string)  [unwired: 1 in, 2 out]
        n260 = Decimal String To Number(string=w578) -> (number=w573:i32)  [unwired: 2 in, 1 out]
        n261 = Fract/Exp String To Number(string=w564) -> (number=w574:dbl)  [unwired: 3 in, 1 out]
        n262 = call "Move Absolute.vi"("error in (no error)"=w576, "Position (0 units)"=w574, "Axis (1)"=w573, "VISA resource name"=w575) -> ("error out"=w571:errorcluster, "VISA resource name out"=w572:refnum<visa-resource-name>)  [unwired: 2 in]
        n263 = case shown="\"wait\"" w563 {
          tunnel: w573 -> [_ w589]
          tunnel: w572 -> [w581 w588]
          tunnel: w571 -> [w580 w587]
          tunnel: [w581 w586] -> w570
          tunnel: [w580 w584] -> w568
          tunnel: w567 -> [_ w583]
          frame "", Default {
          }
          frame "wait" {
            n264 = while {
              tunnel: w589 -> [w595]
              shift-right: [w592] -> w586
              shift-left: w588 -> [w594]
              shift-right: [w591] -> w585
              shift-left: w587 -> [w593]
              stop <- w590 stop-if-true
              n265 = call "Get Axis Motion Status.vi"("error in (no error)"=w593, "Axis (1)"=w595, "VISA resource name"=w594) -> ("error out"=w591:errorcluster, "Motion Done"=w590:bool, "VISA resource name out"=w592:refnum<visa-resource-name>)  [unwired: 2 in]
            }
            n266 = Enqueue Element(queue=w583, element="done", error in (no error)=w585) -> (error out=w584:errorcluster)  [unwired: 1 in, 2 out]
          }
        }
      }
      frame "suspend" {
        n267 = Dequeue Element(queue=w599) -> ()  [unwired: 2 in, 4 out]
      }
      frame "release" {
        n268 = Dequeue Element(queue=w600) -> ()  [unwired: 2 in, 4 out]
        n269 = call "Close.vi"("VISA resource name"=w603) -> ("error out"=w602:errorcluster)  [unwired: 10 in]
      }
      frame "close" {
        n270 = Release Queue(queue=w607) -> ()  [unwired: 2 in, 3 out]
      }
      frame "init" {
        n271 = Dequeue Element(queue=w612) -> ()  [unwired: 2 in, 4 out]
        n272 = flat-sequence {
          tunnel: [w615] -> w609
          tunnel: [w614] -> w608
          tunnel: [w619] -> w610
          tunnel: [w620] -> w611
          tunnel: w609 -> [w620]
          tunnel: w608 -> [w619]
          frame #0 {
            n273 = local write "ESP_con?"(FALSE ("ESP_con?")) -> ()
          }
          frame #1 {
            n274 = call "Initialize.vi"("VISA resource name"="ESP301 VISA", "Serial Link (RS232)"=enum16{"RS232", "USB"}."USB") -> ("VISA resource name out"=w615:refnum<visa-resource-name>, "error out"=w614:errorcluster)  [unwired: 7 in]
          }
          frame #2 {
            n275 = local write "ESP_con?"(TRUE ("ESP_con?")) -> ()
          }
        }
      }
    }
  }
  n276 = while {
    tunnel: w20 -> [w628]
    shift-right: [w626] -> _
    shift-left: _ -> [w624]
    shift-right: [w625] -> _
    shift-left: _ -> [w623]
    shift-right: [w621] -> _
    shift-left: 0 -> [w622]
    stop <- w627 stop-if-true
    n277 = Preview Queue Element(queue=w628, timeout in ms (-1)=w622) -> (queue out=w631:refnum<queue>, element=w632:string)  [unwired: 1 in, 2 out]
    n278 = Match Pattern(string=w632, regular expression=":") -> (before substring=w630:string, after substring=w629:string)  [unwired: 1 in, 2 out]
    n279 = case shown="\"idle\", Default" w630 {
      tunnel: w631 -> [_ _ w649 w653 w662 w673]
      tunnel: w629 -> [_ _ _ _ _ _]
      tunnel: [_ _ _ _ TRUE _] -> w627
      tunnel: [w635 w637 w651 refnum<k5> refnum ("gateway_connection out") w660 w664] -> w626
      tunnel: [w634 w636 w650 w655 w659 w663] -> w625
      tunnel: w624 -> [w635 w637 w651 w657 w660 _]
      tunnel: w623 -> [w634 w636 w650 _ w659 _]
      tunnel: [_ _ -1 _ _ _] -> w621
      frame "idle", Default {
      }
      frame "relative" {
        n280 = disable-structure shown="Disabled" {
          frame Disabled {
            n281 = case shown="True" FALSE {
              tunnel: [_ w647] -> w639
              frame False {
              }
              frame True {
                n282 = call "sp_manip_get_axis_status.vi"("gateway_connection"=w647) -> ("error out"=w642:errorcluster, "axis_out"=w646:T6, "gateway_connection out"=w640:refnum<k5>)  [unwired: 6 in, 2 out]
                n283 = Index Array(array=w646) -> (element=w645:T7, index=w648:i32)
                n284 = Unbundle By Name(w645) -> ("Axis_Name"=w641:string)  [unwired: 1 out]
                n285 = Build Array(w641) -> (w644:string[])
                n286 = Build Array() -> (w643:void[])  [unwired: 1 in]
                n287 = call "sp_manip_start_move.vi"("error in"=w642, "target positions"=w643, "axis names"=w644, "gateway_connection"=w640) -> ()  [unwired: 4 in, 4 out]
              }
            }
          }
          frame Enabled {
          }
        }
      }
      frame "suspend" {
        n288 = Dequeue Element(queue=w649) -> ()  [unwired: 2 in, 4 out]
      }
      frame "release" {
        n289 = Dequeue Element(queue=w653) -> ()  [unwired: 2 in, 4 out]
        n290 = call "sp_manip_disconnect.vi"("gateway_connection"=w657) -> ("error out"=w656:errorcluster, "gateway_connection_out"=w658:refnum<k5>)  [unwired: 7 in, 2 out]
        n291 = call "tcp_gateway_close_connection.vi"("error in"=w656, "server_connection"=w658) -> ("error out"=w655:errorcluster)  [unwired: 5 in]
      }
      frame "close" {
        n292 = Release Queue(queue=w662) -> ()  [unwired: 2 in, 3 out]
      }
      frame "init" {
        n293 = Dequeue Element(queue=w673) -> ()  [unwired: 2 in, 4 out]
        n294 = call "tcp_gateway_open_connection.vi"() -> ("gateway_connection"=w668:refnum<k5>, "error out"=w667:errorcluster)  [unwired: 5 in, 3 out]
        n295 = call "sp_manip_connect.vi"("error in"=w667, "gateway_connection"=w668) -> ("error out"=w663:errorcluster, "axis_out"=w666:T6, "gateway_connection out"=w664:refnum<k5>)  [unwired: 5 in, 2 out]
        n296 = for {
          tunnel: w666 -> [w676] mode=indexing
          tunnel: [w675] -> w671 mode=indexing
          tunnel: [w674] -> w672 mode=indexing
          n297 = Unbundle By Name(w676) -> ("Axis_Name"=w675:string, "Axis_Position"=w674:dbl)
        }
        "names" <- w671
        "pos" <- w672
        n298 = control-ref of="meas_axis"() -> (w665:refnum<vi>)
        n299 = local write "dest"(w672) -> ()
        n300 = Build Array (concatenate)(w671, "XY") -> (w669:string[])
        n301 = property on="Property Node" class="CmbBox"(reference=w665, "Strings[]"=w669) -> ()  [unwired: 1 in, 2 out]
      }
    }
  }
  n302 = while {
    tunnel: w19 -> [w687]
    shift-right: [w684] -> _
    shift-left: 0 -> [w685]
    shift-right: [w683] -> _
    shift-left: _ -> [w682]
    shift-right: [w681] -> _
    shift-left: _ -> [w680]
    shift-right: [w679] -> _
    shift-left: u32 0 ("pHandle") -> [w678]
    tunnel: string[] ["Kinetic Energy", "Pass Energy", "Coil Current", "Work Function", "Detector Voltage", "Screen Voltage", "Conversion Voltage", "Focus Displacement 1", "Focus Displacement 2"] -> [w677]
    stop <- w686 stop-if-true
    n303 = Preview Queue Element(queue=w687, timeout in ms (-1)=w685) -> (queue out=w690:refnum<queue>, element=w691:string)  [unwired: 1 in, 2 out]
    n304 = Match Pattern(string=w691, regular expression=":") -> (before substring=w689:string, after substring=w688:string)  [unwired: 1 in, 2 out]
    n305 = case shown="\"idle\", Default" w689 {
      tunnel: w690 -> [_ w744 w760 w776 w790 w794 w800]
      tunnel: w688 -> [_ _ _ _ _ _ _]
      tunnel: [_ _ _ _ TRUE _ _] -> w686
      tunnel: [_ _ _ _ _ -1 _] -> w684
      tunnel: [w701 w746 w763 w774 w788 w793 w797] -> w683
      tunnel: w682 -> [w712 w735 w765 w775 w788 w793 _]
      tunnel: [w700 w745 w762 w773 w786 w791 w796] -> w681
      tunnel: w680 -> [w710 w734 w764 _ w786 w791 _]
      tunnel: [w698 w732 w761 w772 w787 w792 w799] -> w679
      tunnel: w678 -> [w698 w732 w761 w771 w787 w792 _]
      tunnel: w677 -> [w699 w725 _ _ _ _ _]
      frame "idle", Default {
        n306 = call "SL2_AD_DLL_Phoibos_GetDeviceState.vi"("dll_path"=w712, "pHandle_in"=w698, "dev_type"=DEF_dev_type."devA (analyzer)", "error in"=w710) -> ("path out"=w697:path, "state"=→"state":T3, "error out"=w696:errorcluster)  [unwired: 2 in]
        n307 = for {
          tunnel: w698 -> [w719]
          tunnel: w699 -> [w717] mode=indexing
          tunnel: [w716] -> w709 mode=indexing
          tunnel: [w715] -> w701
          shift-right: [w714] -> w700
          shift-left: w696 -> [w718]
          tunnel: w697 -> [w713]
          n308 = call "SL2_AD_DLL_Phoibos_GetVoltage.vi"("error in"=w718, "voltage_name"=w717, "pHandle"=w719, "dll path in"=w713) -> ("error out"=w714:errorcluster, "value"=w716:dbl, "dll path out"=w715:path)  [unwired: 3 in]
        }
        n309 = Index Array(array=w709) -> (element #1=→"phoib_I_1":dbl, element #2=→"phoib_I_2":dbl, element #3=→"phoib_I_3":dbl, element #4=→"phoib_I_4":dbl, element #5=→"phoib_I_5":dbl, element #6=→"phoib_I_6":dbl, element #7=→"phoib_I_7":dbl, element #8=→"phoib_I_8":dbl, element #9=→"phoib_I_9":dbl)  [unwired: 9 in]
      }
      frame "set" {
        n310 = Dequeue Element(queue=w744) -> ()  [unwired: 2 in, 4 out]
        n311 = Multiply(x="VoltageRange", y=13) -> (x*y=w741:i32)
        n312 = Add(x="Mode", y=w741) -> (x+y=w738:i32)
        n313 = Index Array(array=u32[] [251749632, 251749633, 251749634, 251749635, 251749636, 251749637, 251749638, 251749639, 251749640, 251749641, 251749642, 251749643, 251749644, 251749645, 251749646, 251749647, 251749648, 251749649, 251749650, 251749651, 251749652, 251749653, 251749654, 251749655, 251749656, 251749657, 251749658, 251749659, 251749660, 251749661, 251749662, 251749663, 251749664, 251749665, 251749666, 251749667, 251749668, 251749669, 251749670, 251749671, 251749672, 251749673, 251749674, 251749675, 251749676, 251749677, 251749678, 251749679, 251749680, 251749681, 251749682, 251749683, 251749684, 251749685, 251749686, 251749687, 251749688, 251749689, 251749690, 251749691, 251749692, 251749693, 251749694, 251749695, 251749696] ("modeIDs"), index=w738) -> (element=w736:u32)
        n314 = Build Array("phoib_I_1s", "phoib_I_2s", "phoib_I_3s", "phoib_I_4s", "phoib_I_5s", "phoib_I_6s", "phoib_I_7s", "phoib_I_8s", "phoib_I_9s") -> (w724:dbl[])
        n315 = call "SL2_AD_DLL_Phoibos_SetDeviceMode.vi"("pHandle"=w732, "error in"=w734, "value"=w736, "dev_type"=DEF_dev_type."devA (analyzer)", "dll path in"=w735) -> ("error out"=w723:errorcluster, "dll path out"=w733:path)  [unwired: 4 in]
        n316 = for {
          tunnel: w732 -> [w752]
          shift-right: [w759] -> w746
          shift-left: w733 -> [w756]
          tunnel: w725 -> [w751] mode=indexing
          tunnel: w724 -> [w750] mode=indexing
          shift-right: [w758] -> w745
          shift-left: w723 -> [w754]
          n317 = call "SL2_AD_DLL_Phoibos_GetVoltageRange.vi"("error in"=w754, "voltage_name"=w751, "pHandle"=w752, "dll path in"=w756) -> ("error out"=w753:errorcluster, "min"=w748:dbl, "max"=w749:dbl, "dll path out"=w755:path)  [unwired: 2 in]
          n318 = In Range and Coerce(upper limit=w749, x=w750, lower limit=w748) -> (coerced(x)=w747:dbl)  [unwired: 1 out]
          n319 = call "SL2_AD_DLL_Phoibos_SetVoltage.vi"("commit"=TRUE, "pHandle"=w752, "error in"=w753, "value"=w747, "voltageName"=w751, "dll path in"=w755) -> ("error out"=w758:errorcluster, "dll path out"=w759:path)  [unwired: 3 in]
        }
      }
      frame "standby" {
        w766 = T3 0 items=["Off"=-1, "Standby"=0, "On"=1] ("state")
        n320 = Dequeue Element(queue=w760) -> ()  [unwired: 2 in, 4 out]
        n321 = call "SL2_AD_DLL_Phoibos_SetDeviceState.vi"("pHandle_in"=w761, "error in"=w764, "state"=w766, "dev_type"=DEF_dev_type."devA (analyzer)", "dll_path"=w765) -> ("error out"=w762:errorcluster, "path out"=w763:path)  [unwired: 2 in]
      }
      frame "release" {
        n322 = Dequeue Element(queue=w776) -> ()  [unwired: 2 in, 4 out]
        n323 = flat-sequence {
          tunnel: w775 -> [w777]
          tunnel: w771 -> [w778]
          tunnel: [w781] -> w770
          tunnel: [w780] -> w769
          tunnel: [u32 0] -> w768
          tunnel: [w783] -> w772
          tunnel: [w784] -> w773
          tunnel: [w785] -> w774
          tunnel: w770 -> [w785]
          tunnel: w769 -> [w784]
          tunnel: w768 -> [w783]
          frame #0 {
            n324 = call "SL2_AD_DLL_Phoibos_Shutdown.vi"("pHandle"=w778, "dll path in"=w777) -> ("error out"=w780:errorcluster, "dll path out"=w781:path)  [unwired: 4 in]
          }
          frame #1 {
            n325 = local write "phoib_con?"(FALSE ("phoib_con?")) -> ()
          }
        }
      }
      frame "close" {
        n326 = Release Queue(queue=w790) -> ()  [unwired: 2 in, 3 out]
      }
      frame "suspend" {
        n327 = Dequeue Element(queue=w794) -> ()  [unwired: 2 in, 4 out]
      }
      frame "init" {
        n328 = Dequeue Element(queue=w800) -> ()  [unwired: 2 in, 4 out]
        n329 = flat-sequence {
          tunnel: [w807] -> w798
          tunnel: [w803] -> w797
          tunnel: [w802] -> w796
          tunnel: [w815] -> w799
          tunnel: w798 -> [w815]
          frame #0 {
            n330 = local write "phoib_con?"(FALSE ("phoib_con?")) -> ()
          }
          frame #1 {
            w806 = DEF_dev_type."devA (analyzer)" ("dev_type")
            n331 = call "GetSL2AD_VI_dllPath.vi"() -> ("error"=w810:errorcluster, "Path"=w811:path)  [unwired: 9 in, 1 out]
            n332 = call "SL2_AD_DLL_List_Devices.vi"("error in"=w810, "dev_type"=w806, "dll path in"=w811) -> ("error out"=w804:errorcluster, "devices"=w813:string[], "dll path out"=w805:path)  [unwired: 2 in]
            n333 = Index Array(array=w813) -> (element=w812:string)  [unwired: 1 in]
            n334 = call "SL2_AD_DLL_Phoibos_Initialize.vi"("error in"=w804, "analyzerId"=w812, "dll_path"=w805) -> ("error out"=w808:errorcluster, "pHandle"=w807:u32, "path out"=w809:path)  [unwired: 2 in]
            n335 = call "SL2_AD_DLL_Phoibos_ListDeviceModes.vi"("dll path in"=w809, "dev_type"=w806, "pHandle"=w807, "error in"=w808) -> ("dll path out"=w803:path, "error out"=w802:errorcluster)  [unwired: 1 in, 2 out]
          }
          frame #2 {
            n336 = local write "phoib_con?"(TRUE ("phoib_con?")) -> ()
          }
        }
      }
    }
    "error out 2" <- w681
  }
